vi "FTW-Benchmark-PublisherSubscriber.vi"() -> ()   [LabVIEW 2013]
uses:
  source/actor/Message/Base/FTW-Message.lvclass
  source/actor/Subscriber/FTW-Subscriber.lvclass
  source/actor/Ether/FTW-Ether.lvclass
  source/actor/Publisher/FTW-Publisher.lvclass
panel:
  in  "Wait Time for Workers to Start (ms)":u32=500
  in  "Publishers":i32=8
  in  "Published Message Size":u32=1024
  in  "Publish Period":u32=1
  out "Results":cluster{i32, i32, bool, bool}[](array[cluster])
  in  "Send Timeout":i32=-1
  in  "Send Buffer Depth":i32=-1
  in  "Receive Buffer Depth":i32=-1
  in  "Subscribers":i32=8
  in  "Messages":i32=500
  out "Elapsed Time":dbl format="%.6fsec"
  in  "Connection":string(combo)="inproc://*"
  out "Actual Server Address":string
  out "error out":errorcluster
  # "on slower computers and on the first run, not all pubs may\nbe started by the time the first messages are sent\nincrease this timeout if messages are being lost with lots of\npublishers and lots of subscribers and on slower computers"
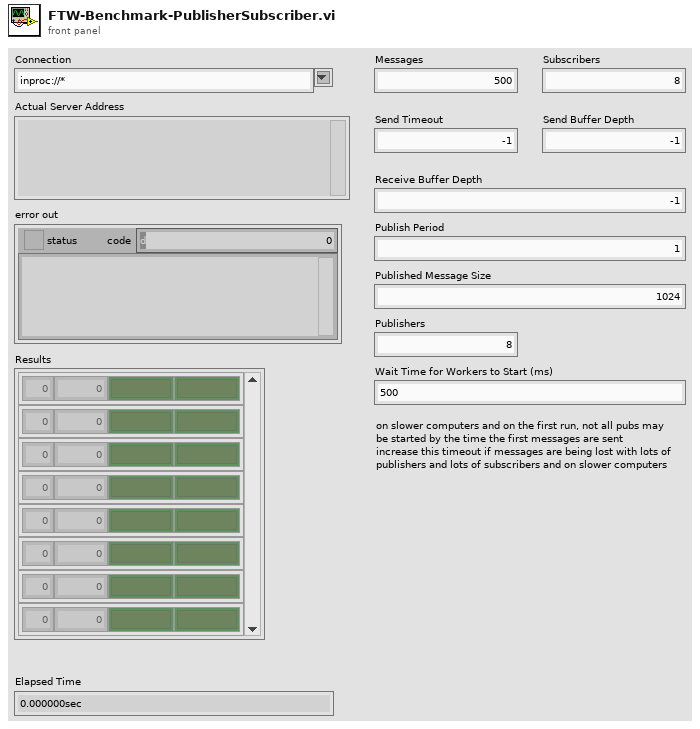
[diagram p1: front panel]
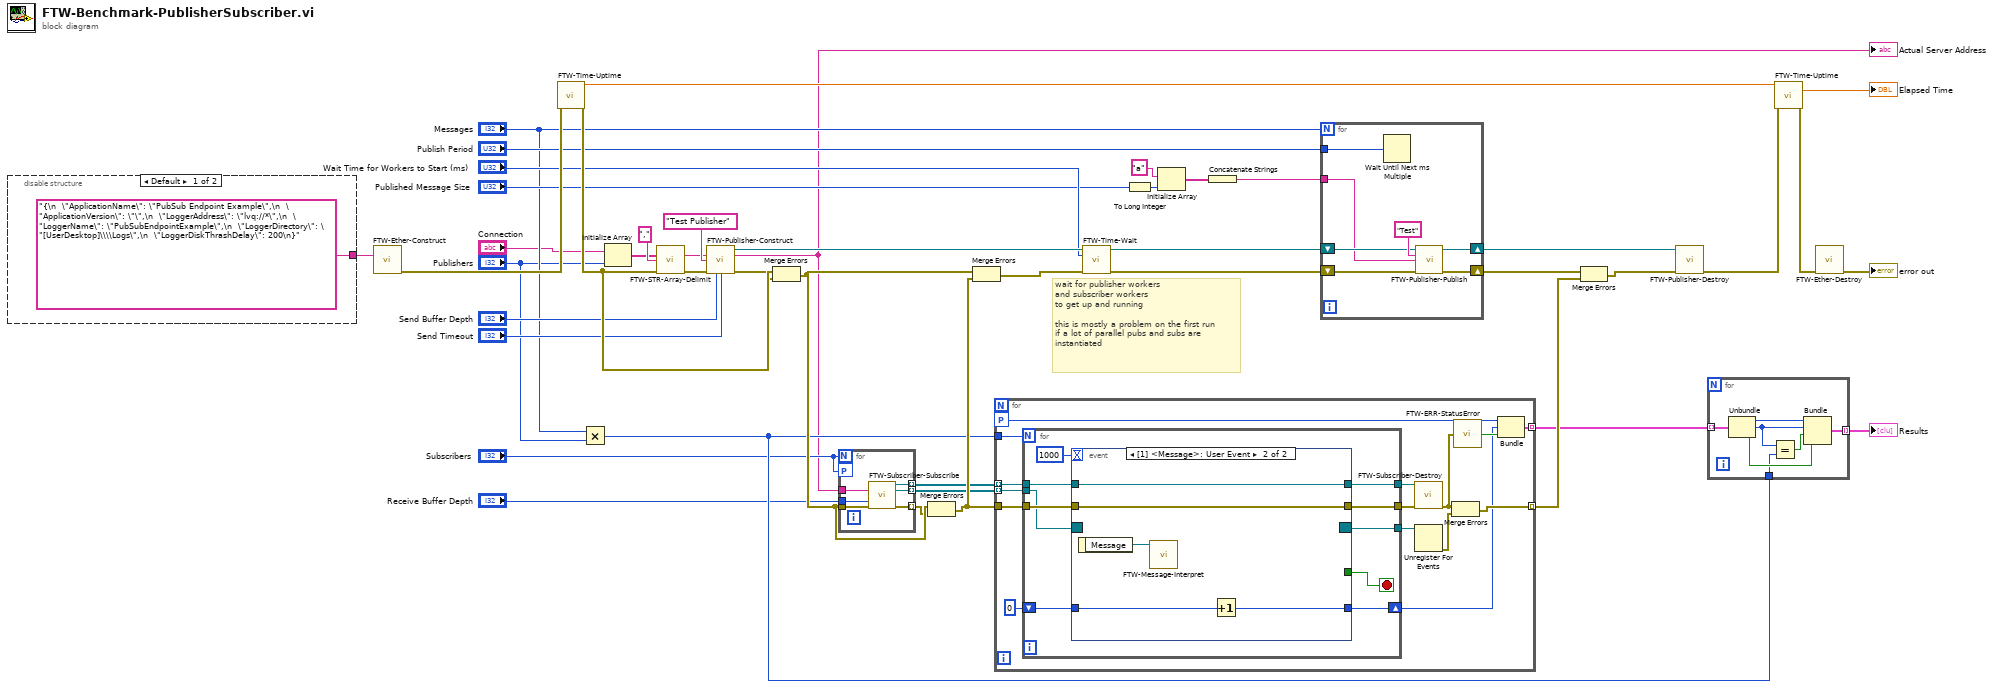
[diagram p0: block diagram]
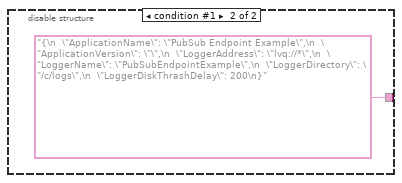
[diagram p2: hidden frame]
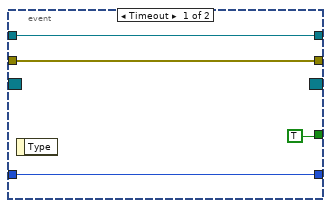
[diagram p3: hidden frame]
diagram:
  # "wait for publisher workers\nand subscriber workers\nto get up and running\n\nthis is mostly a problem on the first run\nif a lot of parallel pubs and subs are\ninstantiated"
  n1 = disable-structure shown="Default" {
    disable-tunnel: ["{\n  \"ApplicationName\": \"PubSub Endpoint Example\",\n  \"ApplicationVersion\": \"\",\n  \"LoggerAddress\": \"lvq://*\",\n  \"LoggerName\": \"PubSubEndpointExample\",\n  \"LoggerDirectory\": \"[UserDesktop]\\\\Logs\",\n  \"LoggerDiskThrashDelay\": 200\n}" ("FTW Ether Configuration") "{\n  \"ApplicationName\": \"PubSub Endpoint Example\",\n  \"ApplicationVersion\": \"\",\n  \"LoggerAddress\": \"lvq://*\",\n  \"LoggerName\": \"PubSubEndpointExample\",\n  \"LoggerDirectory\": \"/c/logs\",\n  \"LoggerDiskThrashDelay\": 200\n}" ("FTW Ether Configuration")] -> w12
    frame condition #0 (active) {
    }
    frame condition #1 {
    }
  }
  n2 = call "FTW-Ether-Construct.vi"("FTW Ether Configuration"=w12) -> ("error out"=w43:errorcluster)  [unwired: 14 in]
  n3 = call "FTW-Time-Uptime.vi"("error in"=w43) -> ("Current Uptime"=w30:dbl, "error out"=w41:errorcluster)  [unwired: 12 in, 1 out]
  n4 = Multiply(x="Messages", y="Publishers") -> (x*y=w13:i32)
  n5 = Initialize Array("Connection", "Publishers") -> (w2:string[])
  n6 = call "FTW-STR-Array-Delimit.vi"("Array of Strings"=w2, "Delimiter"=",") -> ("Delimited String"=w3:string)  [unwired: 13 in]
  n7 = call "FTW-Publisher-Construct.vi"("Address"=w3, "Identity"="Test Publisher", "error in"=w41, "Send Buffer Depth (1)"="Send Buffer Depth", "Send Timeout (-1)"="Send Timeout") -> ("FTW-Publisher Out"=w35:refnum<class "FTW-Publisher.lvclass">, "Actual Address"=w1:string, "error out"=w28:errorcluster)  [unwired: 8 in]
  "Actual Server Address" <- w1
  n8 = Merge Errors(w41, w28) -> (w40:errorcluster)
  n9 = for {
    N: "Subscribers" -> [_]
    tunnel: w40 -> [w51]
    tunnel: [w50] -> w11 mode=indexing
    tunnel: "Receive Buffer Depth" -> [w49]
    tunnel: w1 -> [w48]
    workers-P: "Subscribers" -> [_]
    tunnel: [w47] -> w8 mode=indexing
    tunnel: [w46] -> w7 mode=indexing
    n10 = call "FTW-Subscriber-Subscribe.vi"("Addresses"=w48, "Buffer Depth (1 element)"=w49, "error in"=w51) -> ("FTW-Subscription Out"=w47:refnum<class "FTW-Subscriber.lvclass">, "Subscriber Registration"=w46:refnum<event-registration>, "error out"=w50:errorcluster)  [unwired: 10 in]
  }
  n11 = Merge Errors(w40, w11) -> (w38:errorcluster)
  n12 = Merge Errors(w40, w38) -> (w39:errorcluster)
  n13 = for {
    tunnel: w38 -> [w66]
    tunnel: [w62] -> w25 mode=indexing
    workers-P: _ -> [w60]
    tunnel: [w57] -> w24 mode=indexing
    tunnel: w13 -> [w54]
    tunnel: w8 -> [w53] mode=indexing
    tunnel: w7 -> [w52] mode=indexing
    n14 = for {
      N: w54 -> [_]
      tunnel: w52 -> [w75]
      tunnel: w53 -> [w74]
      tunnel: w66 -> [w76]
      tunnel: [w73] -> w65
      tunnel: [w72] -> w64
      tunnel: [w70] -> w63
      shift-right: [w67] -> w55
      shift-left: 0 -> [w68]
      stop <- w69 stop-if-true
      n15 = event shown="[1] <Message>: User Event" {
        selector: w75 -> [_ _]
        dyn-events: [_ _] -> w70
        timeout: 1000 -> [_ _]
        tunnel: w74 -> [w80 w84]
        tunnel: w76 -> [w79 w83]
        tunnel: [w80 w84] -> w73
        tunnel: [w79 w83] -> w72
        tunnel: [TRUE _] -> w69
        tunnel: [w77 w81] -> w67
        tunnel: w68 -> [w77 w82]
        event Timeout {
          n16 = event-data() -> ()  [unwired: 1 in, 1 out]
        }
        event User Event {
          n17 = event-data() -> ("Message"=w85:refnum<class "FTW-Message.lvclass">)  [unwired: 1 in]
          n18 = call-dynamic "FTW-Message-Interpret.vi"("FTW Message"=w85) -> ()  [unwired: 10 in, 5 out]
          n19 = Increment(x=w82) -> (x+1=w81:i32)
        }
      }
    }
    n20 = call "FTW-Subscriber-Destroy.vi"("FTW-Subscription In"=w65, "error in"=w64) -> ("error out"=w59:errorcluster)  [unwired: 13 in]
    n21 = Unregister For Events(event registration refnum=w63) -> (error out=w61:errorcluster)  [unwired: 1 in]
    n22 = Merge Errors(w59, w61) -> (w62:errorcluster)
    n23 = call "FTW-ERR-StatusError.vi"("error to check"=w59) -> ("Error?"=w58:bool)
    n24 = Bundle(w60, w55, "Error?"=w58) -> (w57:cluster{i32, i32, "Error?":bool})  [unwired: 1 in]
  }
  n25 = call "FTW-Time-Wait.vi"("Wait Time (ms)"="Wait Time for Workers to Start (ms)", "error in"=w39) -> ("error out"=w42:errorcluster)  [unwired: 13 in]
  n26 = To Long Integer(number="Published Message Size") -> (32bit integer=w20:i32)
  n27 = Initialize Array("a", w20) -> (w18:string[])
  n28 = Concatenate Strings(w18) -> (w17:string)
  n29 = for {
    N: "Messages" -> [_]
    tunnel: "Publish Period" -> [w87]
    shift-right: [w89] -> w33
    shift-left: w35 -> [w90]
    shift-right: [w91] -> w36
    shift-left: w42 -> [w88]
    tunnel: w17 -> [w86]
    n30 = Wait Until Next ms Multiple(millisecond multiple=w87) -> ()  [unwired: 1 out]
    n31 = call "FTW-Publisher-Publish.vi"("FTW-Publisher In"=w90, "Header"="Test" ("Message Header"), "Body"=w86, "error in"=w88) -> ("FTW-Publisher Out"=w89:refnum<class "FTW-Publisher.lvclass">, "error out"=w91:errorcluster)  [unwired: 10 in]
  }
  n32 = Merge Errors(w36, w25) -> (w15:errorcluster)
  n33 = call "FTW-Publisher-Destroy.vi"("FTW-Publisher In"=w33, "error in"=w15) -> ("error out"=w34:errorcluster)  [unwired: 13 in]
  n34 = for {
    tunnel: w24 -> [w99] mode=indexing
    tunnel: [w97] -> w23 mode=indexing
    tunnel: w13 -> [w93]
    n35 = Unbundle(w99) -> (w98:i32, w94:i32, "Error?"=w95:bool)
    n36 = Equal?(x=w94, y=w93) -> (x = y?=w96:bool)
    n37 = Bundle(w98, w94, w96, "Error?"=w95) -> (w97:cluster{i32, i32, bool, "Error?":bool})  [unwired: 1 in]
  }
  "Results" <- w23
  n38 = call "FTW-Time-Uptime.vi"("Previous Uptime"=w30, "error in"=w34) -> ("Elapsed Time"=→"Elapsed Time":dbl, "error out"=w31:errorcluster)  [unwired: 11 in, 1 out]
  n39 = call "FTW-Ether-Destroy.vi"("error in"=w31) -> ("error out"=→"error out":errorcluster)  [unwired: 14 in]
